vi "Sub Initialize.vi"(8 "error in (no error)":errorcluster, 11 "Instrument Recorder in":refnum<class "Resonance Detector.lvclass">) -> (0 "error out":errorcluster, 2 "Initialize Result":refnum<class "Acquired Result.lvclass">, 3 "Instrument Recorder out":refnum<class "Resonance Detector.lvclass">)   [LabVIEW 2018, in "Resonance Detector.lvclass"]
uses:
  Resonance Detector.lvclass
  C:/github/LabActor/Process Object/Process Object.lvclass
  NHMFL_Core/Libraries/Instruments/Results/Acquired Result/Acquired Result.lvclass
  Process Object/Process Object.lvclass/Process Object.ctl
  Process Object/Write Broadcaster name.vi
  Read Line detector configuration.vi
  Process Object/Process Object.lvclass
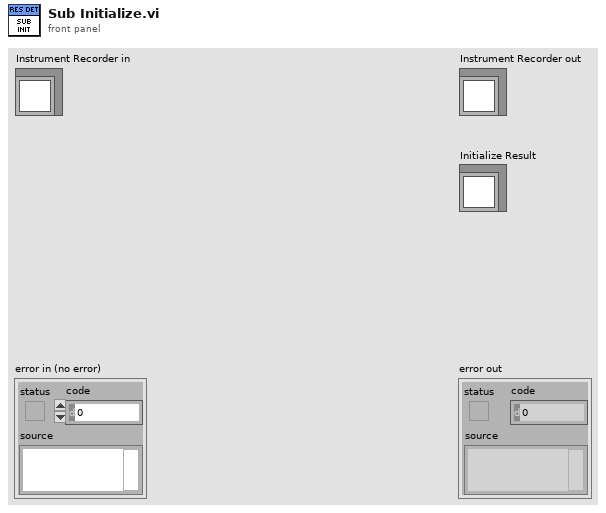
[diagram p1: front panel]
types:
  T1 = typedef "Line Detector Configuration.ctl" = cluster{"Peak width guess":dbl, "Background removal":enum16{"NONE", "High-pass", "Detrend"}, "Smoothing":enum16{"NONE", "Low-pass", "Denoise"}, "Smooth window":dbl, "Relative threshold":dbl, "Finder algorithm":enum16{"Basic", "Wavelet", "Wavelet+detrend"}, "Bgd window":dbl, "Spectrum recorder module name":string, "Fit window":dbl, "Initial fit guess":enum16{"Peak finder", "Last fit"}, "Follow\npeaks":bool, "Re-sample":dbl}
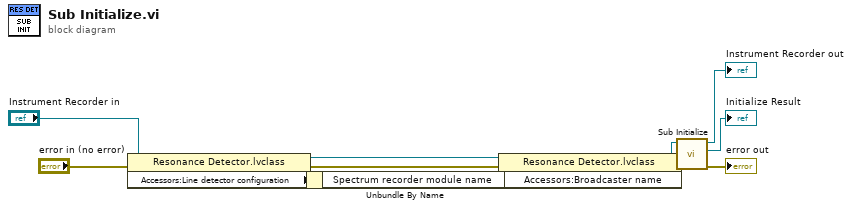
[diagram p0: block diagram]
diagram:
  n1 = property class="Resonance Detector.lvclass"(reference="Instrument Recorder in", error in="error in (no error)") -> (reference out=w8:refnum<class "Resonance Detector.lvclass">, error out=w6:errorcluster, "Accessors:Line detector configuration"=w10:T1)
  n2 = Unbundle By Name(w10) -> ("Spectrum recorder module name"=w7:string)
  n3 = property class="Resonance Detector.lvclass"(reference=w8, error in=w6, "Accessors:Broadcaster name"=w7) -> (reference out=w5:refnum<class "Resonance Detector.lvclass">, error out=w3:errorcluster)
  n4 = call-parent "Sub Initialize.vi"("error in (no error)"=w3, "Measure Object in"=w5) -> ("error out"=→"error out":errorcluster, "Initialize Result"=→"Initialize Result":refnum<class "Acquired Result.lvclass">, "Measure Object out"=→"Instrument Recorder out":refnum<class "Resonance Detector.lvclass">)  [unwired: 7 in]
